vi "Hall_analysis.vi"(4 "interpolation size":u16 min=1 step=1, 5 "max H":sgl=2.0 min=0 format="%.2f", 9 "data worksheet":string="2.000E+0\t-9.081E-1\t\n2.000E+0\t-9.082E-1\t\n2.000E+0\t-9.083E-1\t\n2.000E+0\t-9.081E-1\t\n2.000E+0\t-9.083E-1\t\n1.750E+0\t-9.075E-1\t\n1.750E+0\t-9.076E-1\t\n1.750E+0\t-9.073E-1\t\n1.750E+0\t-9.075E-1\t\n1.750E+0\t-9.075E-1\t\n1.500E+0\t-9.067E-1\t\n1.500E+0\t-9.068E-1\t\n1.500E+0\t-9.067E-1\t\n1.500E+0\t-9.067E-1\t\n1.500E+0\t-9.067E-1\t\n1.250E+0\t-9.057E-1\t\n1.250E+0\t-9.060E-1\t\n1.250E+0\t-9.059E-1\t\n1.250E+0\t-9.059E-1\t\n1.250E+0\t-9.057E-1\t\n1.000E+0\t-9.109E-1\t\n1.000E+0\t-9.109E-1\t\n1.000E+0\t-9.109E-1\t\n1.000E+0\t-9.108E-1\t\n1.000E+0\t-9.109E-1\t\n7.500E-1\t-9.041E-1\t\n7.500E-1\t-9.042E-1\t\n7.500E-1\t-9.042E-1\t\n7.500E-1\t-9.042E-1\t\n7.500E-1\t-9.042E-1\t\n5.000E-1\t-9.032E-1\t\n5.000E-1\t-9.031E-1\t\n2.000E+0\t-9.086E-1\t\n1.890E+0\t-9.080E-1\t\n1.780E+0\t-9.078E-1\t\n1.670E+0\t-9.074E-1\t\n1.560E+0\t-9.070E-1\t\n1.450E+0\t-9.068E-1\t\n1.340E+0\t-9.121E-1\t\n1.230E+0\t-9.058E-1\t\n1.120E+0\t-9.054E-1\t\n1.010E+0\t-9.111E-1\t\n9.000E-1\t-9.048E-1\t\n7.900E-1\t-9.044E-1\t\n6.800E-1\t-9.038E-1\t\n6.300E-1\t-9.037E-1\t\n5.800E-1\t-9.037E-1\t\n5.300E-1\t-9.033E-1\t\n4.800E-1\t-9.034E-1\t\n4.300E-1\t-9.029E-1\t\n3.800E-1\t-9.029E-1\t\n3.300E-1\t-9.043E-1\t\n2.800E-1\t-9.059E-1\t\n2.300E-1\t-9.135E-1\t\n1.800E-1\t-9.091E-1\t\n1.300E-1\t-9.108E-1\t\n8.000E-2\t-9.123E-1\t\n0.000E+0\t-9.211E-1\t") -> (1 "y(x)":cluster{"all rows":dbl[], "smoothed":dbl[]}[](graph)=[{"all rows"=[0.0, 0.08, 0.13, 0.18, 0.23, 0.28, 0.33, 0.38, 0.43, 0.48, 0.5, 0.5, 0.53, 0.58, 0.63, 0.68, 0.75, 0.75, 0.75, 0.75, 0.75, 0.79, 0.9, 1.0, 1.0, 1.0, 1.0, 1.0, 1.01, 1.12, 1.23, 1.25, 1.25, 1.25, 1.25, 1.25, 1.34, 1.45, 1.5, 1.5, 1.5, 1.5, 1.5, 1.56, 1.67, 1.75, 1.75, 1.75, 1.75, 1.75, 1.78, 1.89, 2.0, 2.0, 2.0, 2.0, 2.0, 2.0], "smoothed"=[-0.9211, -0.9123, -0.9108, -0.9091, -0.9135, -0.9059, -0.9043, -0.9029, -0.9029, -0.9034, -0.9032, -0.9031, -0.9033, -0.9037, -0.9037, -0.9038, -0.9041, -0.9042, -0.9042, -0.9042, -0.9042, -0.9044, -0.9048, -0.9109, -0.9109, -0.9109, -0.9108, -0.9109, -0.9111, -0.9054, -0.9058, -0.9057, -0.906, -0.9059, -0.9059, -0.9057, -0.9121, -0.9068, -0.9067, -0.9068, -0.9067, -0.9067, -0.9067, -0.907, -0.9074, -0.9075, -0.9076, -0.9073, -0.9075, -0.9075, -0.9078, -0.908, -0.9081, -0.9082, -0.9083, -0.9081, -0.9083, -0.9086]}, {"all rows"=[-0.11, -0.22, -0.33, -0.44, -0.55, -0.66, -0.77, -0.88, -0.99, -1.1, -1.21, -1.32, -1.43, -1.54, -1.65, -1.76], "smoothed"=[-0.9188, -0.9289, -0.9264, -0.9297, -0.9303, -0.9307, -0.9309, -0.9314, -0.9378, -0.9319, -0.9324, -0.9329, -0.9393, -0.9335, -0.934, -0.9343]}, {"all rows"=[0.0, 0.08, 0.13, 0.18, 0.23, 0.28, 0.33, 0.38, 0.43, 0.48, 0.5, 0.5, 0.53, 0.58, 0.63, 0.68, 0.75, 0.75, 0.75, 0.75, 0.75, 0.79, 0.9, 1.0, 1.0, 1.0, 1.0, 1.0, 1.01, 1.12, 1.23, 1.25, 1.25, 1.25, 1.25, 1.25, 1.34, 1.45, 1.5, 1.5, 1.5, 1.5, 1.5, 1.56, 1.67, 1.75, 1.75, 1.75, 1.75, 1.75, 1.78, 1.89, 2.0, 2.0, 2.0, 2.0, 2.0, 2.0], "smoothed"=[-0.9211, -0.9123, -0.9108, -0.9091, -0.9135, -0.9059, -0.9043, -0.9029, -0.9029, -0.9034, -0.9032, -0.9031, -0.9033, -0.9037, -0.9037, -0.9038, -0.9041, -0.9042, -0.9042, -0.9042, -0.9042, -0.9044, -0.9048, -0.9109, -0.9109, -0.9109, -0.9108, -0.9109, -0.9111, -0.9054, -0.9058, -0.9057, -0.906, -0.9059, -0.9059, -0.9057, -0.9121, -0.9068, -0.9067, -0.9068, -0.9067, -0.9067, -0.9067, -0.907, -0.9074, -0.9075, -0.9076, -0.9073, -0.9075, -0.9075, -0.9078, -0.908, -0.9081, -0.9082, -0.9083, -0.9081, -0.9083, -0.9086]}, {"all rows"=[-0.11, -0.22, -0.33, -0.44, -0.55, -0.66, -0.77, -0.88, -0.99, -1.1, -1.21, -1.32, -1.43, -1.54, -1.65, -1.76], "smoothed"=[-0.9188, -0.9289, -0.9264, -0.9297, -0.9303, -0.9307, -0.9309, -0.9314, -0.9378, -0.9319, -0.9324, -0.9329, -0.9393, -0.9335, -0.934, -0.9343]}], 3 "Result graph":cluster{"all rows":dbl[], "all rows":dbl[]}[](graph)=[{"all rows"=[0.0, 0.10000000149011612, 0.20000000298023224, 0.30000001192092896, 0.4000000059604645, 0.5, 0.6000000238418579, 0.699999988079071, 0.800000011920929, 0.9000000357627869, 1.0, 1.100000023841858, 1.2000000476837158, 1.3000000715255737, 1.399999976158142, 1.5, 1.600000023841858, 1.7000000476837158, 1.8000000715255737, 1.899999976158142, 2.0], "all rows"=[-0.9211, -0.9116999999552965, -0.9108600002622604, -0.9052599996185303, -0.9029, -0.9032, -0.9037, -0.9038857142346246, -0.9044363636797125, -0.90480000218153, -0.9109, -0.906436362400922, -0.9056909092643044, -0.9092555606418186, -0.909209092057835, -0.9067, -0.9071454546321522, -0.9074375000596047, -0.9078363637664102, -0.9080090908874165, -0.9081]}, {"all rows"=[0.0, 0.10000000149011612, 0.20000000298023224, 0.30000001192092896, 0.4000000059604645, 0.5, 0.6000000238418579, 0.699999988079071, 0.800000011920929, 0.9000000357627869, 1.0, 1.100000023841858, 1.2000000476837158, 1.3000000715255737, 1.399999976158142, 1.5, 1.600000023841858, 1.7000000476837158, 1.8000000715255737, 1.899999976158142, 2.0], "all rows"=[-0.9188, -0.9188, -0.9270636366372759, -0.927081817910888, -0.928500000178814, -0.9300272727272727, -0.9304818182685158, -0.9307727272510529, -0.9310363636905497, -0.9325636384443803, -0.9372636363636363, -0.931900000108372, -0.9323545456712896, -0.9328090912342071, -0.9375545440673828, -0.935609090909091, -0.9337727273810994, -0.9341363637664102, -0.9343, -0.9343, -0.9343]}, {"all rows"=[0.0, 0.10000000149011612, 0.20000000298023224, 0.30000001192092896, 0.4000000059604645, 0.5, 0.6000000238418579, 0.699999988079071, 0.800000011920929, 0.9000000357627869, 1.0, 1.100000023841858, 1.2000000476837158, 1.3000000715255737, 1.399999976158142, 1.5, 1.600000023841858, 1.7000000476837158, 1.8000000715255737, 1.899999976158142, 2.0], "all rows"=[-0.0011500000000000399, 0.003550000022351729, 0.008101818187507714, 0.010910909146178815, 0.01280000008940696, 0.01341363636363635, 0.013390909134257944, 0.013443506508214131, 0.013300000005418589, 0.013881818131425139, 0.013181818181818128, 0.012731818853725041, 0.013331818203492607, 0.011776765296194258, 0.014172726004773928, 0.014454545454545498, 0.01331363637447358, 0.01334943185340276, 0.013231818116794913, 0.013145454556291736, 0.0131]}, {"all rows"=[0.0], "all rows"=[]}])   [LabVIEW 2020]
uses:
  <vilib>/Utility/file.llb/Read Delimited Spreadsheet (DBL).vi
  <vilib>/Analysis/NI_AALPro.lvlib
  <vilib>/gmath/NI_Gmath.lvlib
panel:
  out "size(s)":i32
  out "data":dbl[][](array[numeric])=[[0.0, 0.08, 0.13, 0.18, 0.23, 0.28, 0.33, 0.38, 0.43, 0.48, 0.5, 0.5, 0.53, 0.58, 0.63, 0.68, 0.75, 0.75, 0.75, 0.75, 0.75, 0.79, 0.9, 1.0, 1.0, 1.0, 1.0, 1.0, 1.01, 1.12, 1.23, 1.25, 1.25, 1.25, 1.25, 1.25, 1.34, 1.45, 1.5, 1.5, 1.5, 1.5, 1.5, 1.56, 1.67, 1.75, 1.75, 1.75, 1.75, 1.75, 1.78, 1.89, 2.0, 2.0, 2.0, 2.0, 2.0, 2.0], [-0.9211, -0.9123, -0.9108, -0.9091, -0.9135, -0.9059, -0.9043, -0.9029, -0.9029, -0.9034, -0.9032, -0.9031, -0.9033, -0.9037, -0.9037, -0.9038, -0.9041, -0.9042, -0.9042, -0.9042, -0.9042, -0.9044, -0.9048, -0.9109, -0.9109, -0.9109, -0.9108, -0.9109, -0.9111, -0.9054, -0.9058, -0.9057, -0.906, -0.9059, -0.9059, -0.9057, -0.9121, -0.9068, -0.9067, -0.9068, -0.9067, -0.9067, -0.9067, -0.907, -0.9074, -0.9075, -0.9076, -0.9073, -0.9075, -0.9075, -0.9078, -0.908, -0.9081, -0.9082, -0.9083, -0.9081, -0.9083, -0.9086]]
  in  "Negative sweep data file":path
  in  "Full or Positive sweep data file":path=path "C:/work/data/PPMS/FeGaTe312_TC_THE_10K3"
  in  "Reload data file":bool
  in  "Data analyis method":T1(ring)
  in  "field region":dbl[](array[numeric])
  out "slope and residue":string="NaN\tNaN"
  out "linear fit high":dbl
  out "linear fit low":dbl
  out "slope":dbl=nan format="%#.6g"
  out "residue":dbl=nan format="%#.6g"
  in  "method":u16(ring) items=["Least Square", "Least Absolute Residual", "Bisquare"]
  in  "iteration Number":i32=2
  in  "smooth factor":i32=121
  in  "smooth":bool
  out "Field, RawData, Field_int, Hall":string="-1.76000E+0\t-9.34300E-1\t0.00000E+0\t-1.15000E-3\r\n-1.65000E+0\t-9.34000E-1\t1.00000E-1\t3.55000E-3\r\n-1.54000E+0\t-9.33500E-1\t2.00000E-1\t8.10182E-3\r\n-1.43000E+0\t-9.39300E-1\t3.00000E-1\t1.09109E-2\r\n-1.32000E+0\t-9.32900E-1\t4.00000E-1\t1.28000E-2\r\n-1.21000E+0\t-9.32400E-1\t5.00000E-1\t1.34136E-2\r\n-1.10000E+0\t-9.31900E-1\t6.00000E-1\t1.33909E-2\r\n-9.90000E-1\t-9.37800E-1\t7.00000E-1\t1.34435E-2\r\n-8.80000E-1\t-9.31400E-1\t8.00000E-1\t1.33000E-2\r\n-7.70000E-1\t-9.30900E-1\t9.00000E-1\t1.38818E-2\r\n-6.60000E-1\t-9.30700E-1\t1.00000E+0\t1.31818E-2\r\n-5.50000E-1\t-9.30300E-1\t1.10000E+0\t1.27318E-2\r\n-4.40000E-1\t-9.29700E-1\t1.20000E+0\t1.33318E-2\r\n-3.30000E-1\t-9.26400E-1\t1.30000E+0\t1.17768E-2\r\n-2.20000E-1\t-9.28900E-1\t1.40000E+0\t1.41727E-2\r\n-1.10000E-1\t-9.18800E-1\t1.50000E+0\t1.44545E-2\r\n0.00000E+0\t-9.21100E-1\t1.60000E+0\t1.33136E-2\r\n8.00000E-2\t-9.12300E-1\t1.70000E+0\t1.33494E-2\r\n1.30000E-1\t-9.10800E-1\t1.80000E+0\t1.32318E-2\r\n1.80000E-1\t-9.09100E-1\t1.90000E+0\t1.31455E-2\r\n2.30000E-1\t-9.13500E-1\t2.00000E+0\t1.31000E-2\r\n2.80000E-1\t-9.05900E-1\t0.00000E+0\t0.00000E+0\r\n3.30000E-1\t-9.04300E-1\t0.00000E+0\t0.00000E+0\r\n3.80000E-1\t-9.02900E-1\t0.00000E+0\t0.00000E+0\r\n4.30000E-1\t-9.02900E-1\t0.00000E+0\t0.00000E+0\r\n4.80000E-1\t-9.03400E-1\t0.00000E+0\t0.00000E+0\r\n5.00000E-1\t-9.03200E-1\t0.00000E+0\t0.00000E+0\r\n5.00000E-1\t-9.03100E-1\t0.00000E+0\t0.00000E+0\r\n5.30000E-1\t-9.03300E-1\t0.00000E+0\t0.00000E+0\r\n5.80000E-1\t-9.03700E-1\t0.00000E+0\t0.00000E+0\r\n6.30000E-1\t-9.03700E-1\t0.00000E+0\t0.00000E+0\r\n6.80000E-1\t-9.03800E-1\t0.00000E+0\t0.00000E+0\r\n7.50000E-1\t-9.04100E-1\t0.00000E+0\t0.00000E+0\r\n7.50000E-1\t-9.04200E-1\t0.00000E+0\t0.00000E+0\r\n7.50000E-1\t-9.04200E-1\t0.00000E+0\t0.00000E+0\r\n7.50000E-1\t-9.04200E-1\t0.00000E+0\t0.00000E+0\r\n7.50000E-1\t-9.04200E-1\t0.00000E+0\t0.00000E+0\r\n7.90000E-1\t-9.04400E-1\t0.00000E+0\t0.00000E+0\r\n9.00000E-1\t-9.04800E-1\t0.00000E+0\t0.00000E+0\r\n1.00000E+0\t-9.10900E-1\t0.00000E+0\t0.00000E+0\r\n1.00000E+0\t-9.10900E-1\t0.00000E+0\t0.00000E+0\r\n1.00000E+0\t-9.10900E-1\t0.00000E+0\t0.00000E+0\r\n1.00000E+0\t-9.10800E-1\t0.00000E+0\t0.00000E+0\r\n1.00000E+0\t-9.10900E-1\t0.00000E+0\t0.00000E+0\r\n1.01000E+0\t-9.11100E-1\t0.00000E+0\t0.00000E+0\r\n1.12000E+0\t-9.05400E-1\t0.00000E+0\t0.00000E+0\r\n1.23000E+0\t-9.05800E-1\t0.00000E+0\t0.00000E+0\r\n1.25000E+0\t-9.05700E-1\t0.00000E+0\t0.00000E+0\r\n1.25000E+0\t-9.06000E-1\t0.00000E+0\t0.00000E+0\r\n1.25000E+0\t-9.05900E-1\t0.00000E+0\t0.00000E+0\r\n1.25000E+0\t-9.05900E-1\t0.00000E+0\t0.00000E+0\r\n1.25000E+0\t-9.05700E-1\t0.00000E+0\t0.00000E+0\r\n1.34000E+0\t-9.12100E-1\t0.00000E+0\t0.00000E+0\r\n1.45000E+0\t-9.06800E-1\t0.00000E+0\t0.00000E+0\r\n1.50000E+0\t-9.06700E-1\t0.00000E+0\t0.00000E+0\r\n1.50000E+0\t-9.06800E-1\t0.00000E+0\t0.00000E+0\r\n1.50000E+0\t-9.06700E-1\t0.00000E+0\t0.00000E+0\r\n1.50000E+0\t-9.06700E-1\t0.00000E+0\t0.00000E+0\r\n1.50000E+0\t-9.06700E-1\t0.00000E+0\t0.00000E+0\r\n1.56000E+0\t-9.07000E-1\t0.00000E+0\t0.00000E+0\r\n1.67000E+0\t-9.07400E-1\t0.00000E+0\t0.00000E+0\r\n1.75000E+0\t-9.07500E-1\t0.00000E+0\t0.00000E+0\r\n1.75000E+0\t-9.07600E-1\t0.00000E+0\t0.00000E+0\r\n1.75000E+0\t-9.07300E-1\t0.00000E+0\t0.00000E+0\r\n1.75000E+0\t-9.07500E-1\t0.00000E+0\t0.00000E+0\r\n1.75000E+0\t-9.07500E-1\t0.00000E+0\t0.00000E+0\r\n1.78000E+0\t-9.07800E-1\t0.00000E+0\t0.00000E+0\r\n1.89000E+0\t-9.08000E-1\t0.00000E+0\t0.00000E+0\r\n2.00000E+0\t-9.08100E-1\t0.00000E+0\t0.00000E+0\r\n2.00000E+0\t-9.08200E-1\t0.00000E+0\t0.00000E+0\r\n2.00000E+0\t-9.08300E-1\t0.00000E+0\t0.00000E+0\r\n2.00000E+0\t-9.08100E-1\t0.00000E+0\t0.00000E+0\r\n2.00000E+0\t-9.08300E-1\t0.00000E+0\t0.00000E+0\r\n2.00000E+0\t-9.08600E-1\t0.00000E+0\t0.00000E+0\r\n"
  in  "stop":bool
  in  "offset row":i32=1
  in  "data column":i32=2
  in  "field column":i32
  in  "(1) Data input method":T2(ring)
  # "linear fitting conditions"
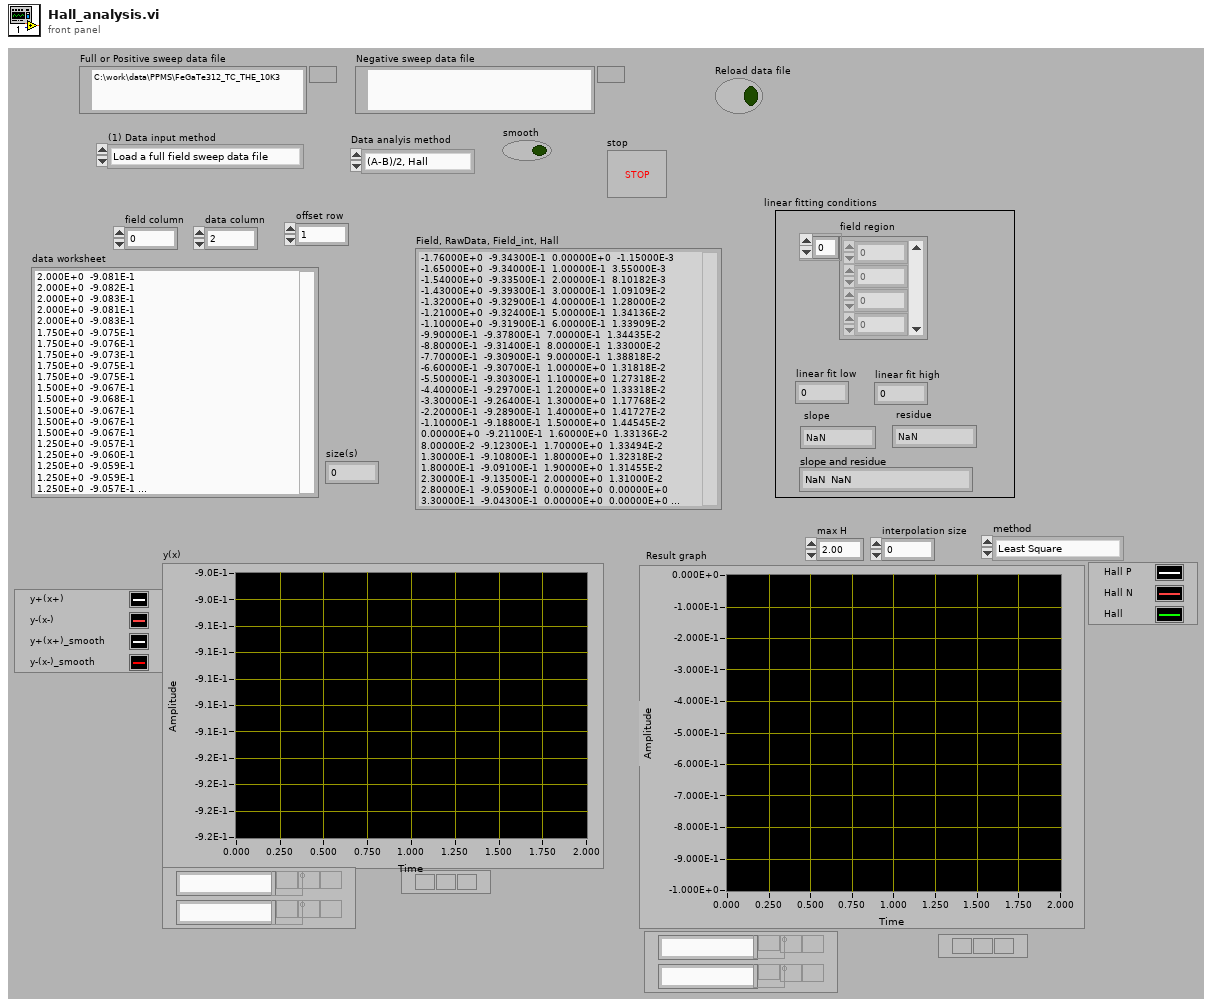
[diagram p1: front panel]
types:
  T1 = enum16{"(A-B)/2, Hall", "(A+B)/2, MR", "diagram defined"}
  T2 = enum16{"Load a full field sweep data file", "Load two seprate sweep data files", "Direct input (copy and paste)"}
  T3 = enum16{"Load a full field sweep data file", "Load two seprate sweep data diles", "Direct input (copy and paste)"}
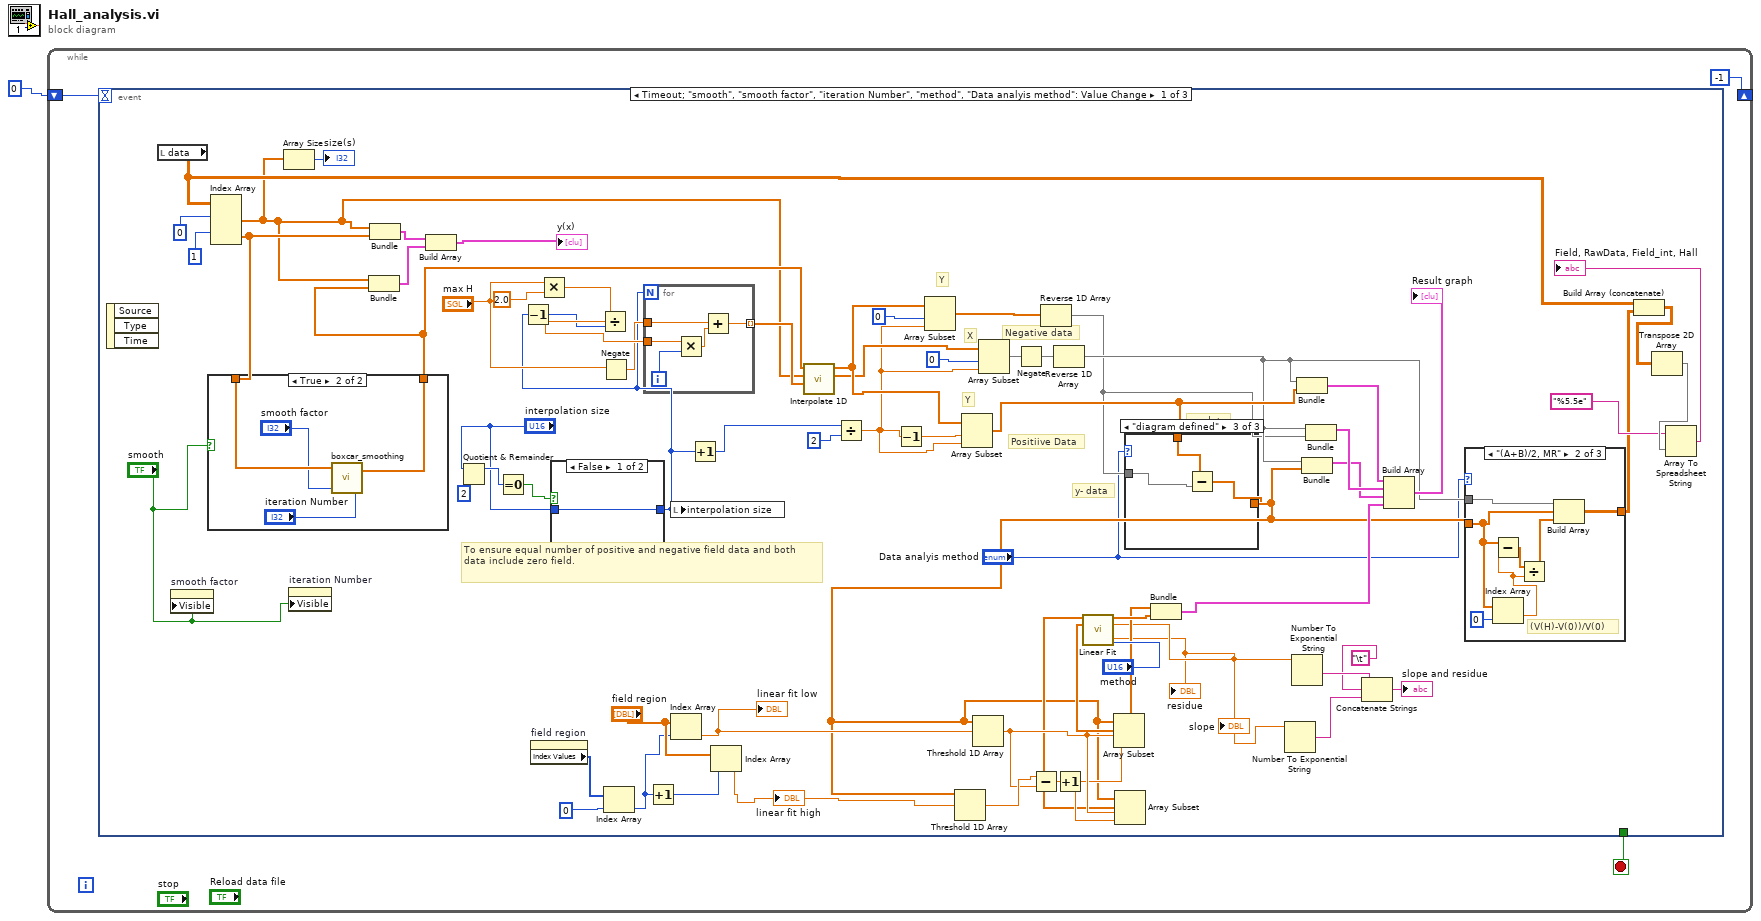
[diagram p0: block diagram]
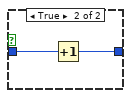
[diagram p2: hidden frame]
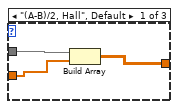
[diagram p3: hidden frame]
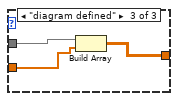
[diagram p4: hidden frame]
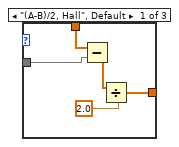
[diagram p5: hidden frame]
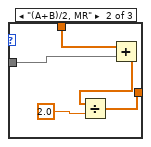
[diagram p6: hidden frame]
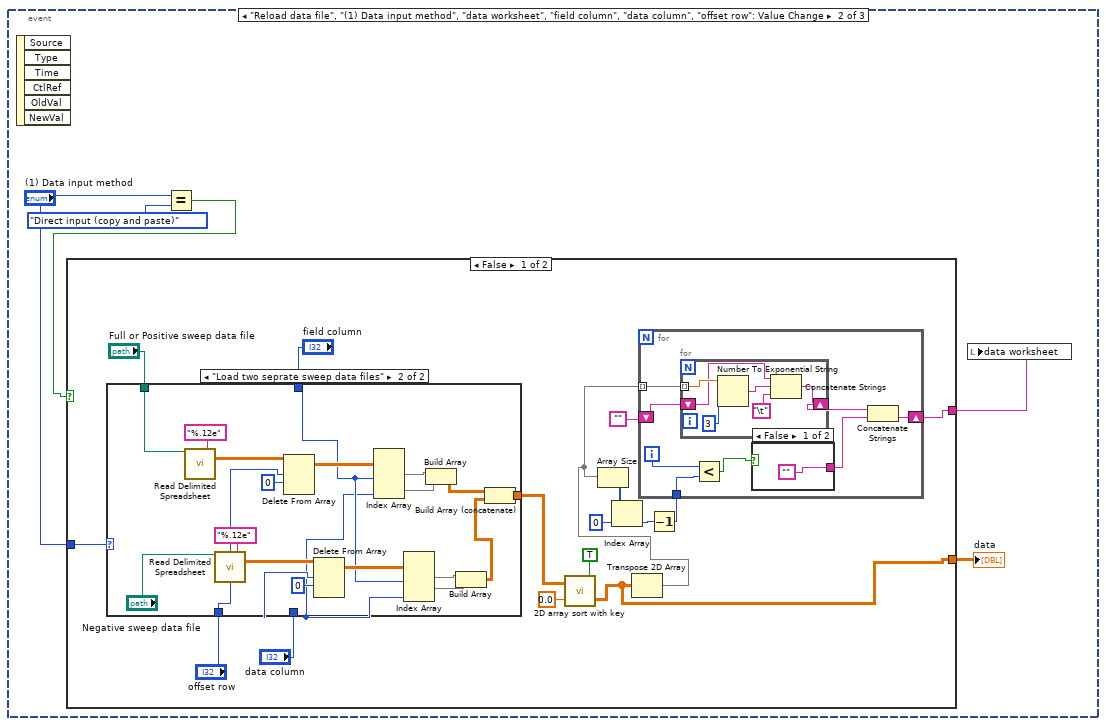
[diagram p8: hidden frame]
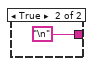
[diagram p9: hidden frame]
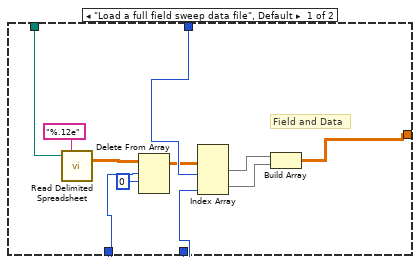
[diagram p10: hidden frame]
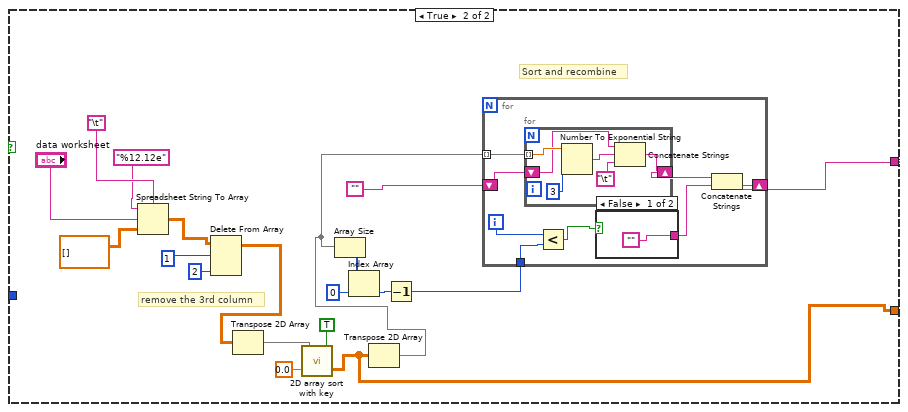
[diagram p11: hidden frame]
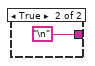
[diagram p12: hidden frame]
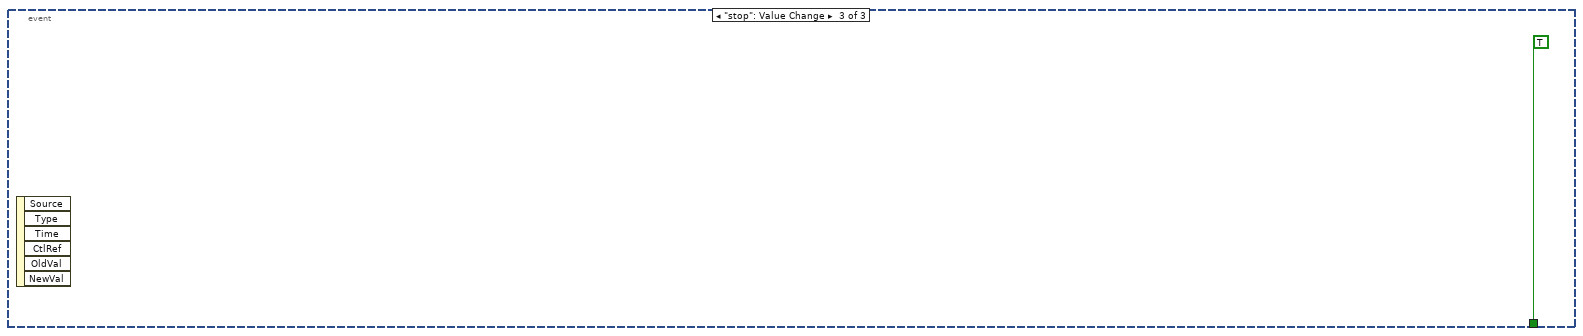
[diagram p13: hidden frame]
diagram:
  n1 = while {
    shift-right: [-1] -> _
    shift-left: 0 -> [w3]
    stop <- w4 stop-if-true
    n2 = event shown="[0] Timeout;  \"smooth\", \"smooth factor\", \"iteration Number\", \"method\", \"Data analyis method\": Value Change" {
      selector: _ -> [_ _ _]
      dyn-events: _ -> [_ _ _]
      timeout: w3 -> [_ _ _]
      tunnel: [_ _ TRUE] -> w4
      event Timeout; "smooth", "smooth factor", "iteration Number", "method", "Data analyis method": Value Change {
        # "y- data"
        # "Y"
        # "X"
        # "Y"
        # "Negative data"
        # "Positiive Data"
        # "To ensure equal number of positive and negative field data and both\ndata include zero field."
        # "y+ data"
        n3 = event-data() -> ()  [unwired: 1 in, 3 out]
        n4 = local read "data"() -> (w8:dbl[][])
        n5 = property on="smooth factor" class="DigNum (strict)"("Visible"="smooth") -> ()  [unwired: 2 in, 2 out]
        n6 = Index Array(array=w8, index (row) #1=0 ("disabled index (col)"), index (row) #2=1 ("index (col)")) -> (element #1=w6:dbl[], element #2=w44:dbl[])  [unwired: 2 in]
        n7 = case shown="True" "smooth" {
          tunnel: w44 -> [w109 w113]
          tunnel: [w109 w112] -> w31
          frame False {
          }
          frame True {
            n8 = call "boxcar_smoothing.vi"("iteration Number"="iteration Number", "smooth factor"="smooth factor", "raw data"=w113) -> ("smoothed"=w112:dbl[])  [unwired: 1 in]
          }
        }
        n9 = Array Size(array=w6) -> (size(s)=→"size(s)":i32)
        n10 = property on="iteration Number" class="DigNum (strict)"("Visible"="smooth") -> ()  [unwired: 2 in, 2 out]
        n11 = Bundle("data"=w6, "smoothed"=w31) -> (w38:cluster{" data":dbl[], "smoothed":dbl[]})  [unwired: 1 out]
        n12 = Bundle("data"=w6, "data"=w44) -> (w9:cluster{" data":dbl[], " data":dbl[]})  [unwired: 1 out]
        n13 = Build Array(w9, w38) -> (→"y(x)":cluster{" data":dbl[], "smoothed":dbl[]}[])
        n14 = Quotient & Remainder(x="interpolation size", y=u16 2) -> (x-y*floor(x/y)=w24:u16)  [unwired: 1 out]
        n15 = Equal To 0?(x=w24) -> (x = 0?=w25:bool)
        n16 = property on="field region" class="Arr (strict)"() -> ("Index Values"=w49:u32[])  [unwired: 2 in, 2 out]
        n17 = Multiply(x="max H", y=sgl 2.0) -> (x*y=w36:sgl)
        n18 = case shown="False" w25 {
          tunnel: "interpolation size" -> [w75 w77]
          tunnel: [w75 w76] -> w23
          frame False {
          }
          frame True {
            n19 = Increment(x=w77) -> (x+1=w76:u16)
          }
        }
        n20 = Decrement(x=w23) -> (x-1=w10:u16)
        n21 = Divide(x=w36, y=w10) -> (x/y=w35:sgl)
        n22 = Negate(x="max H") -> (-x=w33:sgl)
        n23 = Index Array(array=w49, index=0) -> (element=w47:u32)
        n24 = for {
          N: w23 -> [_]
          tunnel: w35 -> [w81]
          tunnel: w33 -> [w79]
          tunnel: [w78] -> w32 mode=indexing
          i -> [w82]
          n25 = Multiply(x=w81, y=w82) -> (x*y=w80:sgl)
          n26 = Add(x=w79, y=w80) -> (x+y=w78:sgl)
        }
        n27 = Increment(x=w47) -> (x+1=w52:u32)
        n28 = local write "interpolation size"(w23) -> ()
        n29 = Index Array(array="field region", index=w47) -> (element=w51:dbl)
        "linear fit low" <- w51
        n30 = Increment(x=w23) -> (x+1=w22:u16)
        n31 = Index Array(array="field region", index=w52) -> (element=w50:dbl)
        "linear fit high" <- w50
        n32 = call <vilib>:"Interpolate 1D.vi"("xi"=w32, "X"=w6, "Y"=w31) -> ("xi used"=w21:dbl[], "yi"=w27:dbl[])  [unwired: 6 in, 1 out]
        n33 = Divide(x=w22, y=u16 2) -> (x/y=w19:dbl)
        n34 = Decrement(x=w19) -> (x-1=w20:dbl)
        n35 = Array Subset(array=w27, index=0, length=w19) -> (w17:dbl[])
        n36 = Array Subset(array=w27, index=w20, length=w19) -> (w15:dbl[])
        n37 = Array Subset(array=w21, index=0, length=w19) -> (w18:dbl[])
        n38 = Negate(x=w18) -> (-x=w16:dbl[])
        n39 = Reverse 1D Array(array=w17) -> (reversed array=w13:dbl[])
        n40 = Reverse 1D Array(array=w16) -> (reversed array=w14:dbl[])
        n41 = case shown="\"diagram defined\"" "Data analyis method" {
          tunnel: w15 -> [w100 w105 w108]
          tunnel: w13 -> [w97 w102 w107]
          tunnel: [w96 w101 w106] -> w12
          frame "(A-B)/2, Hall", Default {
            n42 = Subtract(x=w100, y=w97) -> (x-y=w98:dbl[])
            n43 = Divide(x=w98, y=2.0) -> (x/y=w96:dbl[])
          }
          frame "(A+B)/2, MR" {
            n44 = Add(x=w105, y=w102) -> (x+y=w103:dbl[])
            n45 = Divide(x=w103, y=2.0) -> (x/y=w101:dbl[])
          }
          frame "diagram defined" {
            n46 = Subtract(x=w108, y=w107) -> (x-y=w106:dbl[])
          }
        }
        n47 = Threshold 1D Array(2:w50, 3:w12) -> (0:w65:dbl)  [unwired: 1 out]
        n48 = Threshold 1D Array(2:w51, 3:w12) -> (0:w63:dbl)  [unwired: 1 out]
        n49 = Subtract(x=w65, y=w63) -> (x-y=w64:dbl)
        n50 = Increment(x=w64) -> (x+1=w62:dbl)
        n51 = Array Subset(array=w12, index=w63, length=w62) -> (w60:dbl[])
        n52 = Array Subset(array=w12, index=w63, length=w62) -> (w61:dbl[])
        n53 = call <vilib>:"Linear Fit.vi"("Y"=w61, "X"=w60, "method"="method") -> ("Best Linear Fit"=w66:dbl[], "slope"=w59:dbl, "residue"=w57:dbl)  [unwired: 3 in, 7 out]
        "residue" <- w57
        "slope" <- w59
        n54 = Bundle(w60, "Best Linear Fit"=w66) -> (w67:cluster{dbl[], "Best Linear Fit":dbl[]})  [unwired: 1 out]
        n55 = Number To Exponential String(number=w57) -> (E-format string=w55:string)  [unwired: 3 out]
        n56 = Number To Exponential String(number=w59) -> (E-format string=w58:string)  [unwired: 3 out]
        n57 = Bundle(w14, w15) -> (w74:cluster{dbl[], dbl[]})  [unwired: 1 out]
        n58 = Bundle(w14, w12) -> (w72:cluster{dbl[], dbl[]})  [unwired: 1 out]
        n59 = Bundle(w14, w13) -> (w73:cluster{dbl[], dbl[]})  [unwired: 1 out]
        n60 = Concatenate Strings(w58, "\t", w55) -> (→"slope and residue":string)
        n61 = Build Array(w74, w73, w72, w67) -> (→"Result graph":cluster{dbl[], "Best Linear Fit":dbl[]}[])
        n62 = case shown="\"(A+B)/2, MR\"" "Data analyis method" {
          tunnel: [w85 w87 w95] -> w40
          tunnel: w14 -> [w84 w92 w94]
          tunnel: w12 -> [w83 w90 w93]
          frame "(A-B)/2, Hall", Default {
            n63 = Build Array(w84, w83) -> (w85:dbl[][])
          }
          frame "(A+B)/2, MR" {
            # "(V(H)-V(0))/V(0)"
            n64 = Index Array(array=w90, index=0) -> (element=w88:dbl)
            n65 = Subtract(x=w90, y=w88) -> (x-y=w91:dbl[])
            n66 = Divide(x=w91, y=w88) -> (x/y=w86:dbl[])
            n67 = Build Array(w92, w90, w86) -> (w87:dbl[][])
          }
          frame "diagram defined" {
            n68 = Build Array(w94, w93) -> (w95:dbl[][])
          }
        }
        n69 = Build Array (concatenate)(w8, w40) -> (w39:dbl[][])
        n70 = Transpose 2D Array(2D array=w39) -> (transposed array=w70:dbl[][])
        n71 = Array To Spreadsheet String(array=w70, 3:"%5.5e" ("format string")) -> (spreadsheet string=→"Field, RawData, Field_int, Hall":string)  [unwired: 1 out]
      }
      event "Reload data file", "(1) Data input method", "data worksheet", "field column", "data column", "offset row": Value Change {
        n72 = event-data() -> ()  [unwired: 1 in, 6 out]
        n73 = Equal?(x="(1) Data input method", y=T3."Direct input (copy and paste)") -> (x = y?=w117:bool)
        n74 = case shown="False" w117 {
          tunnel: [w121 w186] -> w115
          tunnel: "(1) Data input method" -> [w125 _]
          tunnel: [w119 w184] -> w114
          frame False {
            n75 = case shown="\"Load two seprate sweep data files\"" w125 {
              tunnel: "field column" -> [w161 w166]
              tunnel: "data column" -> [w160 w165]
              tunnel: "offset row" -> [w159 w167]
              tunnel: "Full or Positive sweep data file" -> [w158 w169]
              tunnel: [w151 w162] -> w122
              frame "Load a full field sweep data file", Default {
                # "Field and Data"
                n76 = call-poly <vilib>:"Read Delimited Spreadsheet.vi"("file path (dialog if empty)"=w158, "format (%.3f)"="%.12e") -> ("all rows"=w156:dbl[][])  [unwired: 8 in, 5 out]
                n77 = Delete From Array(array=w156, length=w159, index (row)=0) -> (array with subset deleted=w154:dbl[][])  [unwired: 1 in, 1 out]
                n78 = Index Array(array=w154, index (col) #1=w161, index (col) #2=w160) -> (element #1=w153:dbl[], element #2=w152:dbl[])  [unwired: 2 in]
                n79 = Build Array(w153, w152) -> (w151:dbl[][])
              }
              frame "Load two seprate sweep data files" {
                n80 = call-poly <vilib>:"Read Delimited Spreadsheet.vi"("file path (dialog if empty)"=w169, "format (%.3f)"="%.12e") -> ("all rows"=w177:dbl[][])  [unwired: 8 in, 5 out]
                n81 = call-poly <vilib>:"Read Delimited Spreadsheet.vi"("file path (dialog if empty)"="Negative sweep data file", "format (%.3f)"="%.12e") -> ("all rows"=w171:dbl[][])  [unwired: 8 in, 5 out]
                n82 = Delete From Array(array=w177, length=w167, index (row)=0) -> (array with subset deleted=w176:dbl[][])  [unwired: 1 in, 1 out]
                n83 = Delete From Array(array=w171, length=w167, index (row)=0) -> (array with subset deleted=w170:dbl[][])  [unwired: 1 in, 1 out]
                n84 = Index Array(array=w176, index (col) #1=w166, index (col) #2=w165) -> (element #1=w180:dbl[], element #2=w179:dbl[])  [unwired: 2 in]
                n85 = Index Array(array=w170, index (col) #1=w166, index (col) #2=w165) -> (element #1=w174:dbl[], element #2=w173:dbl[])  [unwired: 2 in]
                n86 = Build Array(w180, w179) -> (w164:dbl[][])
                n87 = Build Array(w174, w173) -> (w163:dbl[][])
                n88 = Build Array (concatenate)(w164, w163) -> (w162:dbl[][])
              }
            }
            n89 = call "2D array sort with key.vi"("ascending"=TRUE, "key row"=0.0, "input"=w122) -> ("output"=w119:dbl[][])
            n90 = Transpose 2D Array(2D array=w119) -> (transposed array=w120:dbl[][])
            n91 = Array Size(array=w120) -> (size(s)=w129:i32[])
            n92 = Index Array(array=w129, index=0) -> (element=w127:i32)
            n93 = Decrement(x=w127) -> (x-1=w126:i32)
            n94 = for {
              tunnel: w120 -> [w142] mode=indexing
              shift-right: [w140] -> w121
              shift-left: "" -> [w139]
              tunnel: w126 -> [w135]
              i -> [w137]
              n95 = for {
                tunnel: w142 -> [w150] mode=indexing
                shift-right: [w146] -> w141
                shift-left: w139 -> [w147]
                n96 = Number To Exponential String(number=w150, precision (6)=i16 3) -> (E-format string=w148:string)  [unwired: 2 in]
                n97 = Concatenate Strings(w147, w148, "\t") -> (w146:string)
              }
              n98 = Less?(x=w137, y=w135) -> (x < y?=w136:bool)
              n99 = case shown="False" w136 {
                tunnel: ["" "\n"] -> w138
                frame False {
                }
                frame True {
                }
              }
              n100 = Concatenate Strings(w141, w138) -> (w140:string)
            }
          }
          frame True {
            # "Sort and recombine"
            # "remove the 3rd column"
            n101 = Spreadsheet String To Array(delimiter (Tab)="\t", format string="%12.12e", spreadsheet string="data worksheet", array type (2D Dbl)=dbl[][] []) -> (array=w194:dbl[][])
            n102 = Delete From Array(array=w194, length=1, index (col)=2 ("disabled index (col)")) -> (array with subset deleted=w183:dbl[][])  [unwired: 1 in, 1 out]
            n103 = Transpose 2D Array(2D array=w183) -> (transposed array=w182:dbl[][])
            n104 = call "2D array sort with key.vi"("ascending"=TRUE, "key row"=0.0, "input"=w182) -> ("output"=w184:dbl[][])
            n105 = Transpose 2D Array(2D array=w184) -> (transposed array=w185:dbl[][])
            n106 = Array Size(array=w185) -> (size(s)=w192:i32[])
            n107 = Index Array(array=w192, index=0) -> (element=w190:i32)
            n108 = Decrement(x=w190) -> (x-1=w189:i32)
            n109 = for {
              tunnel: w185 -> [w208] mode=indexing
              shift-right: [w206] -> w186
              shift-left: "" -> [w205]
              tunnel: w189 -> [w201]
              i -> [w203]
              n110 = for {
                tunnel: w208 -> [w216] mode=indexing
                shift-right: [w212] -> w207
                shift-left: w205 -> [w213]
                n111 = Number To Exponential String(number=w216, precision (6)=i16 3) -> (E-format string=w214:string)  [unwired: 2 in]
                n112 = Concatenate Strings(w213, w214, "\t") -> (w212:string)
              }
              n113 = Less?(x=w203, y=w201) -> (x < y?=w202:bool)
              n114 = case shown="False" w202 {
                tunnel: ["" "\n"] -> w204
                frame False {
                }
                frame True {
                }
              }
              n115 = Concatenate Strings(w207, w204) -> (w206:string)
            }
          }
        }
        "data" <- w114
        n116 = local write "data worksheet"(w115) -> ()
      }
      event "stop": Value Change {
        n117 = event-data() -> ()  [unwired: 1 in, 6 out]
      }
    }
  }
